vi "ErrorHandler.vi"(6 "Instance":i32, 8 "error in (no error)":errorcluster, 11 "Msg":string) -> (0 "error out":errorcluster)   [LabVIEW 2017, in "Communication.lvlib"]
uses:
  Communication.lvlib
  MsgError.ctl
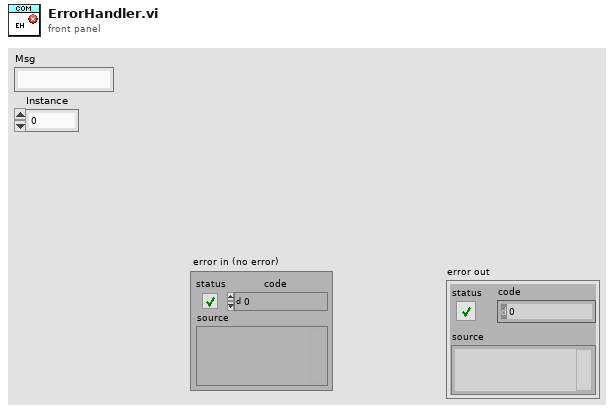
[diagram p1: front panel]
types:
  T1 = typedef "Communication.lvlib/MsgError.ctl" = cluster{"error in (no error)":errorcluster, "Msg":string}
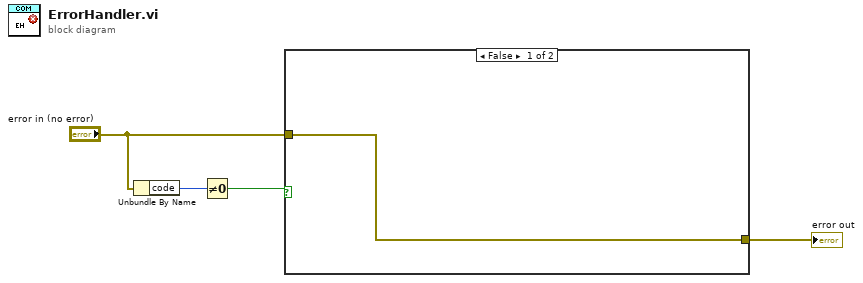
[diagram p0: block diagram]
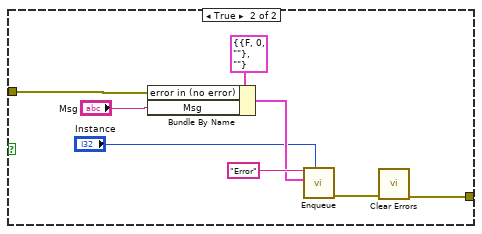
[diagram p2: hidden frame]
diagram:
  n1 = Unbundle By Name("error in (no error)") -> ("code"=w3:i32)
  n2 = Not Equal To 0?(x=w3) -> (x != 0?=w2:bool)
  n3 = case shown="False" w2 {
    tunnel: [w5 w11] -> w4
    tunnel: "error in (no error)" -> [w5 w7]
    frame False {
    }
    frame True {
      n4 = Bundle By Name(cluster=T1 {"error in (no error)"={"status"=FALSE, "code"=0, "source"=""}, "Msg"=""} ("Cluster"), "error in (no error)"=w7, "Msg"="Msg") -> (w8:T1)
      n5 = call "Enqueue.vi"("Instance"="Instance", "Data"=w8, "Msg"="Error") -> ("error out"=w12:errorcluster)  [unwired: 8 in]
      n6 = call <vilib>:"Clear Errors.vi"("error in (no error)"=w12) -> ("error out"=w11:errorcluster)  [unwired: 5 in, 1 out]
    }
  }
  "error out" <- w4
